vi "H Function.vi"(1 "Width":dbl, 2 "Length":dbl) -> (0 "h":dbl)   [LabVIEW 2012]
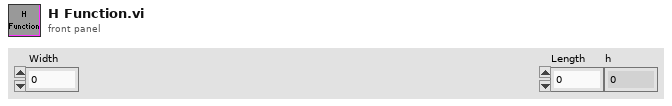
[diagram p1: front panel]
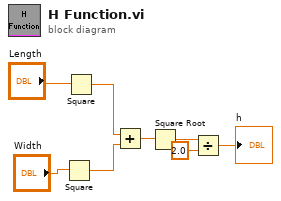
[diagram p0: block diagram]
diagram:
  n1 = Square(x="Width") -> (x^2=w5:dbl)
  n2 = Square(x="Length") -> (x^2=w6:dbl)
  n3 = Add(x=w6, y=w5) -> (x+y=w4:dbl)
  n4 = Square Root(x=w4) -> (sqrt(x)=w3:dbl)
  n5 = Divide(x=w3, y=2.0) -> (x/y=→"h":dbl)
